vi "ReadCalibrationFile(SubVI).vi"(8 "error in (no error)":errorcluster, 11 "appended path":path) -> (0 "error out":errorcluster, 1 "Ch3 WF":dbl[](array[numeric]), 2 "V2":dbl, 3 "V3":dbl, 4 "Ch2 WF":dbl[](array[numeric]), 5 "V1":dbl, 7 "Ch1 WF":dbl[](array[numeric]))   [LabVIEW 2019]
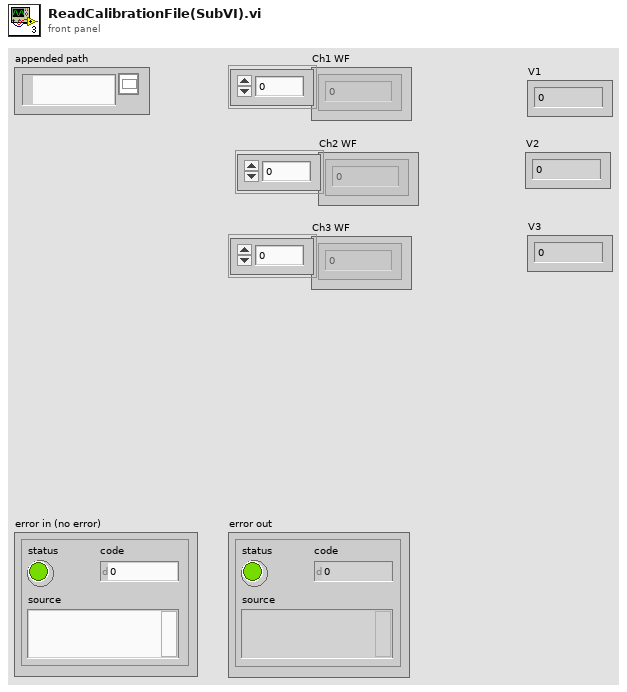
[diagram p1: front panel]
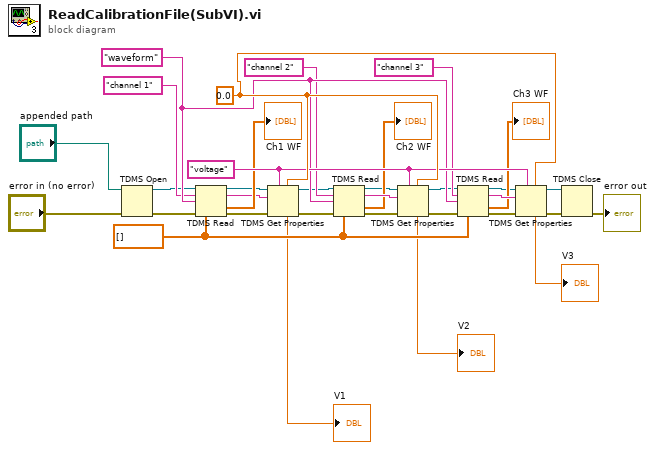
[diagram p0: block diagram]
diagram:
  w32 = 0.0
  w31 = "voltage" ("property name")
  w27 = "waveform" ("channel name(s) in")
  w28 = dbl[] []
  n1 = TDMS Open(8:"error in (no error)", 11:"appended path") -> (0:w3:errorcluster, 3:w2:refnum<k34>)  [unwired: 5 in]
  n2 = TDMS Read(0:w2, 5:"channel 1" ("group name in"), 7:w27, 11:w3, 12:w28) -> (4:w5:refnum<k34>, 6:w7:string, 10:→"Ch1 WF":dbl[], 15:w6:errorcluster)  [unwired: 3 in, 2 out]
  n3 = TDMS Get Properties(5:w32, 7:w31, 8:w6, 10:w7, 11:w5) -> (0:w12:errorcluster, 3:w10:refnum<k34>, 4:→"V1":dbl)  [unwired: 1 in, 3 out]
  n4 = TDMS Read(0:w10, 5:"channel 2" ("group name in"), 7:w27, 11:w12, 12:w28) -> (4:w11:refnum<k34>, 6:w16:string, 10:→"Ch2 WF":dbl[], 15:w13:errorcluster)  [unwired: 3 in, 2 out]
  n5 = TDMS Get Properties(5:w32, 7:w31, 8:w13, 10:w16, 11:w11) -> (0:w19:errorcluster, 3:w18:refnum<k34>, 4:→"V2":dbl)  [unwired: 1 in, 3 out]
  n6 = TDMS Read(0:w18, 5:"channel 3" ("group name in"), 7:w27, 11:w19, 12:w28) -> (4:w20:refnum<k34>, 6:w30:string, 10:→"Ch3 WF":dbl[], 15:w21:errorcluster)  [unwired: 3 in, 2 out]
  n7 = TDMS Get Properties(5:w32, 7:w31, 8:w21, 10:w30, 11:w20) -> (0:w23:errorcluster, 3:w22:refnum<k34>, 4:→"V3":dbl)  [unwired: 1 in, 3 out]
  n8 = TDMS Close(8:w23, 11:w22) -> (0:→"error out":errorcluster)  [unwired: 1 out]
